vi "Interlace.vi"() -> ()   [LabVIEW 2014]
doc: "Use this template to build a VI to use as a subVI."
uses:
  <vilib>/vision/NI_Vision_Development_Module.lvlib
panel:
  out "Frame":T1(plugin-control)
  out "Field":T1(plugin-control)
  # ":: MVi Framework V1.0 ::\nAuthor:Gaoke Yang\nEmail: gaoke.yang@yahoo.com\nWeb: www.mvicontrol.com\nCopyright (C) 2015, MVI Technologies All Rights Reserved"
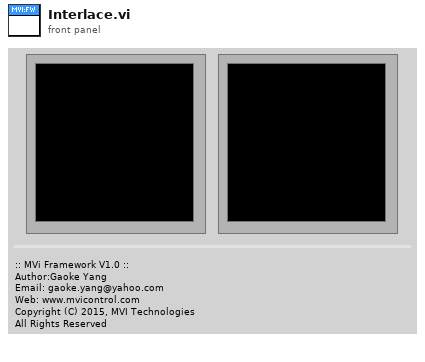
[diagram p1: front panel]
types:
  T1 = typedef "IMAQ Image.ctl" = refnum<image>
  T2 = typedef "Image Type" = u32
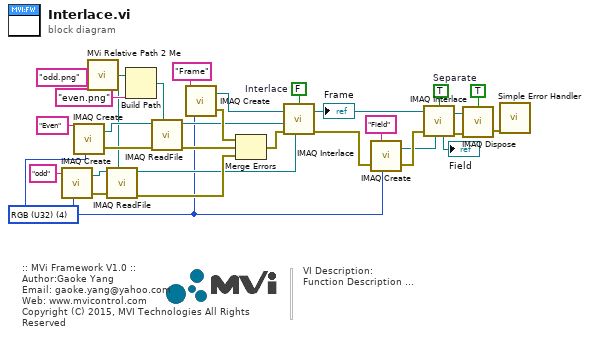
[diagram p0: block diagram]
diagram:
  w9 = TRUE  # Separate
  w27 = FALSE  # Interlace
  w5 = T2 4 items=["Grayscale (U8)", "Grayscale (I16)", "Grayscale (SGL)", "Complex (CSG)", "RGB (U32)", "HSL (U32)", "RGB (U64)", "Grayscale (U16)"] ("Image Type")
  # "VI Description:\nFunction Description ..."
  # ":: MVi Framework V1.0 ::\nAuthor:Gaoke Yang\nEmail: gaoke.yang@yahoo.com\nWeb: www.mvicontrol.com\nCopyright (C) 2015, MVI Technologies All Rights Reserved"
  n1 = call "IMAQ Create"("Image Name"="odd" ("name or relative path"), "Image Type"=w5) -> ("New Image"=w22:T1, "error out"=w23:errorcluster)  [unwired: 2 in, 1 out]
  n2 = call "IMAQ Create"("Image Name"="Even" ("name or relative path"), "Image Type"=w5) -> ("New Image"=w19:T1, "error out"=w20:errorcluster)  [unwired: 2 in, 1 out]
  n3 = call "MVi Relative Path 2 Me.vi"("Relative Path"="odd.png" ("name or relative path")) -> ("Appended Dir"=w12:path, "MyDir"=w21:path)  [unwired: 5 in]
  n4 = call "IMAQ ReadFile"("File Path"=w12, "error in (no error)"=w23, "Image"=w22) -> ("error out"=w18:errorcluster, "Image Out"=w6:T1)  [unwired: 4 in, 3 out]
  n5 = Build Path(base path=w21, name or relative path="even.png") -> (appended path=w26:path)
  n6 = call "IMAQ ReadFile"("File Path"=w26, "error in (no error)"=w20, "Image"=w19) -> ("error out"=w17:errorcluster, "Image Out"=w13:T1)  [unwired: 4 in, 3 out]
  n7 = call "IMAQ Create"("Image Name"="Frame" ("name or relative path"), "Image Type"=w5) -> ("New Image"=w14:T1, "error out"=w16:errorcluster)  [unwired: 2 in, 1 out]
  n8 = Merge Errors(w16, w17, w18) -> (w15:errorcluster)
  n9 = call "IMAQ Interlace"("error in (no error)"=w15, "Image Even"=w13, "Image Odd"=w6, "Image Frame"=w14, "Interlace/Separate (Interlace)"=w27) -> ("error out"=w4:errorcluster, "Image Frame Out"=w8:T1)  [unwired: 2 out]
  "Frame" <- w8
  n10 = call "IMAQ Create"("Image Name"="Field" ("name or relative path"), "Image Type"=w5, "error in (no error)"=w4) -> ("New Image"=w2:T1, "error out"=w3:errorcluster)  [unwired: 1 in, 1 out]
  n11 = call "IMAQ Interlace"("error in (no error)"=w3, "Image Odd"=w2, "Image Frame"=w8, "Interlace/Separate (Interlace)"=w9) -> ("Image Odd Out"=→"Field":T1, "error out"=w10:errorcluster, "Image Frame Out"=w11:T1)  [unwired: 1 in, 1 out]
  n12 = call "IMAQ Dispose"("All Images? (No)"=TRUE, "Image"=w11, "error in (no error)"=w10) -> ("error out"=w29:errorcluster)  [unwired: 3 out]
  n13 = call <vilib>:"Simple Error Handler.vi"("error in (no error)"=w29) -> ()  [unwired: 1 in, 8 out]
